vi "byte24-33 (SubVI).vi"(0 "unsigned byte array":u8[](array[numeric])) -> (1 "Numeric 2":u8, 2 "Numeric":u8, 3 "Numeric 10":u8, 4 "Numeric 9":u8, 6 "Numeric 3":u8, 8 "Numeric 8":u8, 10 "Numeric 7":u8, 12 "Numeric 4":u8, 13 "Numeric 5":u8, 14 "Numeric 6":u8)   [LabVIEW 2016]
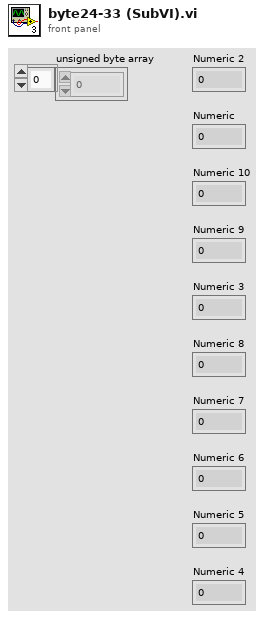
[diagram p1: front panel]
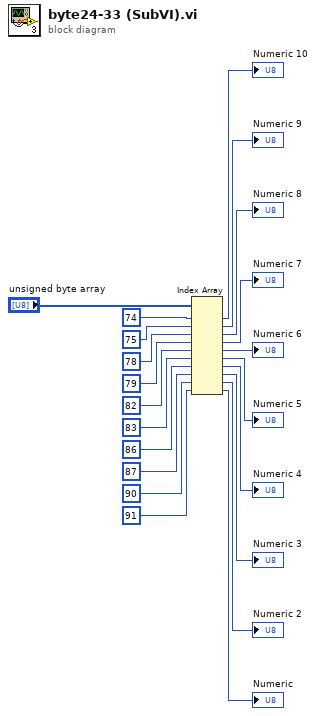
[diagram p0: block diagram]
diagram:
  n1 = Index Array(array="unsigned byte array", index #1=74 ("index"), index #2=75 ("index"), index #3=78 ("index"), index #4=79 ("index"), index #5=82 ("index"), index #6=83 ("index"), index #7=86 ("index"), index #8=87 ("index"), index #9=90 ("index"), index #10=91 ("index")) -> (element #1=→"Numeric 10":u8, element #2=→"Numeric 9":u8, element #3=→"Numeric 8":u8, element #4=→"Numeric 7":u8, element #5=→"Numeric 6":u8, element #6=→"Numeric 5":u8, element #7=→"Numeric 4":u8, element #8=→"Numeric 3":u8, element #9=→"Numeric 2":u8, element #10=→"Numeric":u8)
